vi "generic_test_noTEC.vi"() -> ()   [LabVIEW 2011]
uses:
  C:/OmniDriverSPAM/OOI_HOME/NETOmniDriver-NET20.dll
  OmniDriverSPAM/OOI_HOME/NETOmniDriver-NET20.dll
panel:
  out "getSpectrum Times Array":u32[](array[numeric])
  in  "ExtraDelay\nAfter Loop":bool
  in  "LoopExit":bool
  out "getSpectrumTime [ms]":u32
  in  "Trigger Mode":i32
  out "Spectrometer Type":string
  out "XY Graph":cluster{"Y":dbl[], "Y":dbl[]}[](graph) caption="XY-Graph"
  out "Spectrum":dbl[](array[numeric])
  out "Wavelengths [nm]":dbl[](array[numeric])
  in  "Scans to Average":i32=1
  in  "Int. Time [ms]":i32=1000
  out "MinIntTime [ms]":i32
  out "NETWrapper\nStatus":errorcluster caption="NETWrapper Status"
  out "MaxIntTime [ms]":i32
  in  "spectrometerIndex":i32
  out "Serial\nNumber":string
  out "Number attached\nSpectrometers":i32
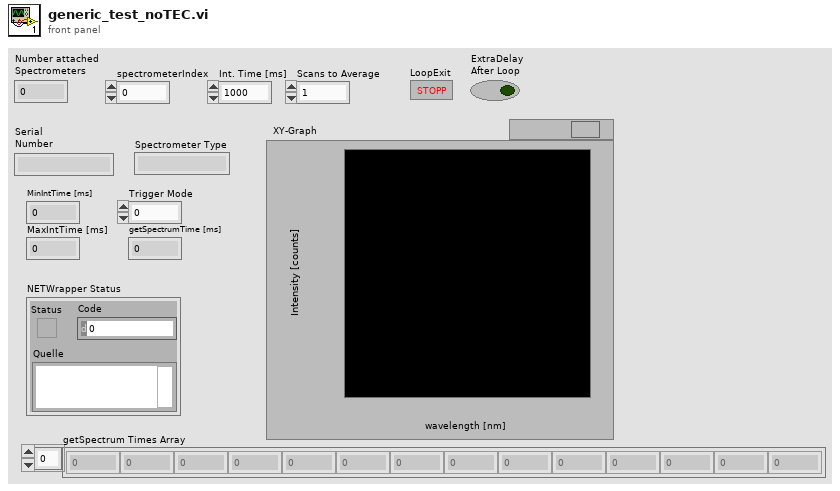
[diagram p1: front panel]
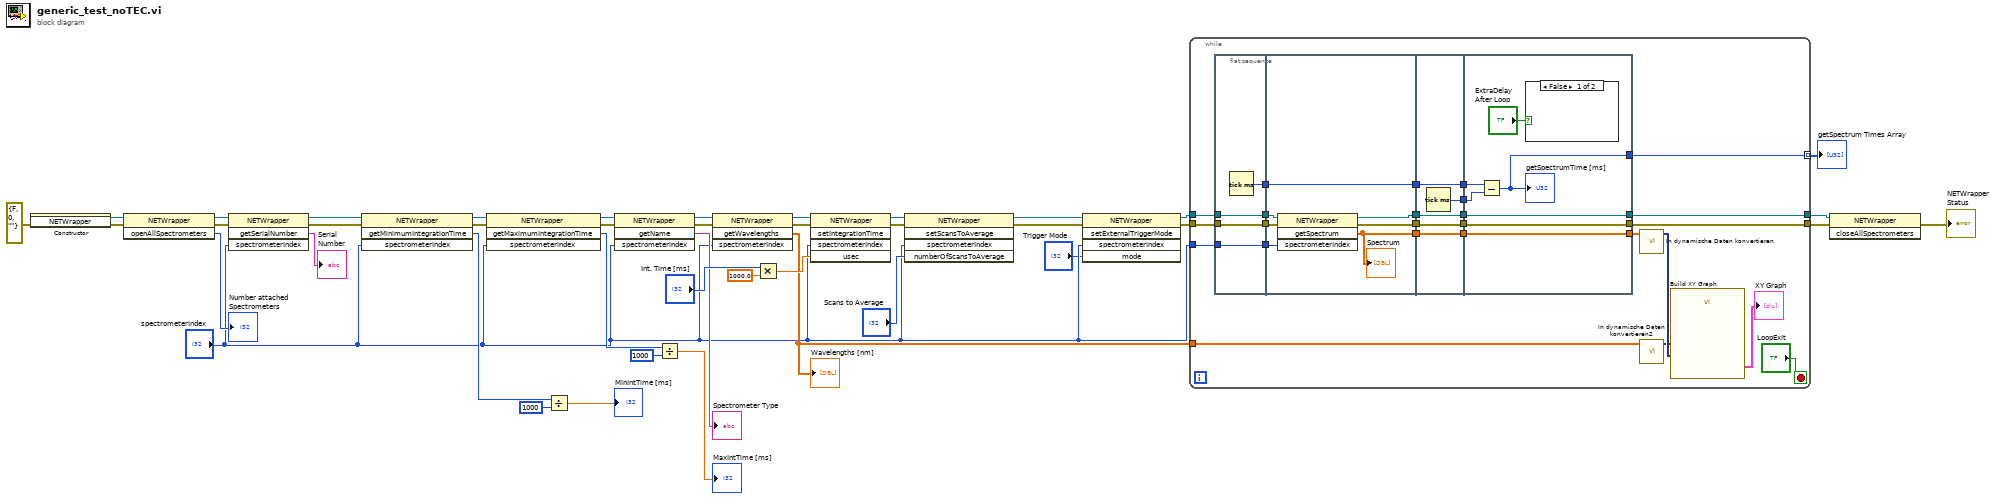
[diagram p0: block diagram]
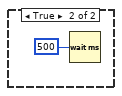
[diagram p2: hidden frame]
diagram:
  n1 = constructor class="NETWrapper"(error in=errorcluster {"status"=FALSE, "code"=0, "source"=""} ("Fehler (Eingang, kein Fehler)")) -> (reference out=w3:refnum<k24>, error out=w2:errorcluster)  [unwired: 2 in, 1 out]
  n2 = invoke class="NETWrapper" method="openAllSpectrometers"(reference=w3, error in=w2) -> (reference out=w40:refnum<k24>, error out=w39:errorcluster, "openAllSpectrometers"=→"Number attached\nSpectrometers":i32)  [unwired: 1 in]
  n3 = invoke class="NETWrapper" method="getSerialNumber"(reference=w40, error in=w39, "spectrometerIndex"="spectrometerIndex") -> (reference out=w37:refnum<k24>, error out=w36:errorcluster, "getSerialNumber"=→"Serial\nNumber":string)  [unwired: 1 in, 1 out]
  n4 = invoke class="NETWrapper" method="getMinimumIntegrationTime"(reference=w37, error in=w36, "spectrometerIndex"="spectrometerIndex") -> (reference out=w35:refnum<k24>, error out=w34:errorcluster, "getMinimumIntegrationTime"=w30:i32)  [unwired: 1 in, 1 out]
  n5 = invoke class="NETWrapper" method="getMaximumIntegrationTime"(reference=w35, error in=w34, "spectrometerIndex"="spectrometerIndex") -> (reference out=w14:refnum<k24>, error out=w16:errorcluster, "getMaximumIntegrationTime"=w15:i32)  [unwired: 1 in, 1 out]
  n6 = Divide(x=w30, y=1000) -> (x/y=→"MinIntTime [ms]":dbl)
  n7 = invoke class="NETWrapper" method="getName"(reference=w14, error in=w16, "spectrometerIndex"="spectrometerIndex") -> (reference out=w12:refnum<k24>, error out=w11:errorcluster, "getName"=→"Spectrometer Type":string)  [unwired: 1 in, 1 out]
  n8 = Divide(x=w15, y=1000) -> (x/y=→"MaxIntTime [ms]":dbl)
  n9 = invoke class="NETWrapper" method="getWavelengths"(reference=w12, error in=w11, "spectrometerIndex"="spectrometerIndex") -> (reference out=w21:refnum<k24>, error out=w20:errorcluster, "getWavelengths"=w17:dbl[])  [unwired: 1 in, 1 out]
  "Wavelengths [nm]" <- w17
  n10 = Multiply(x="Int. Time [ms]", y=1000.0) -> (x*y=w27:dbl)
  n11 = invoke class="NETWrapper" method="setIntegrationTime"(reference=w21, error in=w20, "spectrometerIndex"="spectrometerIndex", "usec"=w27) -> (reference out=w23:refnum<k24>, error out=w24:errorcluster)  [unwired: 1 in, 3 out]
  n12 = invoke class="NETWrapper" method="setScansToAverage"(reference=w23, error in=w24, "spectrometerIndex"="spectrometerIndex", "numberOfScansToAverage"="Scans to Average") -> (reference out=w9:refnum<k24>, error out=w8:errorcluster)  [unwired: 1 in, 3 out]
  n13 = invoke class="NETWrapper" method="setExternalTriggerMode"(reference=w9, error in=w8, "spectrometerIndex"="spectrometerIndex", "mode"="Trigger Mode") -> (reference out=w10:refnum<k24>, error out=w7:errorcluster)  [unwired: 1 in, 3 out]
  n14 = while {
    tunnel: w10 -> [w66]
    tunnel: [w65] -> w19
    tunnel: [w64] -> w18
    tunnel: w17 -> [w60]
    tunnel: "spectrometerIndex" -> [w58]
    tunnel: w7 -> [w57]
    tunnel: [w42] -> w4 mode=indexing
    stop <- "LoopExit" stop-if-true
    n15 = flat-sequence {
      tunnel: w57 -> [w68]
      tunnel: w58 -> [w69]
      tunnel: w66 -> [w70]
      tunnel: [w70] -> w56
      tunnel: [w69] -> w55
      tunnel: [w68] -> w54
      tunnel: [w67] -> w46
      tunnel: w56 -> [w77]
      tunnel: w55 -> [w74]
      tunnel: w54 -> [w73]
      tunnel: [w76] -> w53
      tunnel: [w75] -> w52
      tunnel: [w72] -> w51
      tunnel: w46 -> [w71]
      tunnel: [w71] -> w45
      tunnel: w53 -> [w82]
      tunnel: w52 -> [w81]
      tunnel: w51 -> [w80]
      tunnel: [w82] -> w50
      tunnel: [w81] -> w49
      tunnel: [w80] -> w48
      tunnel: [w79] -> w47
      tunnel: w45 -> [w78]
      tunnel: [w78] -> w44
      tunnel: [w87] -> w62
      tunnel: [w88] -> w64
      tunnel: [w89] -> w65
      tunnel: w50 -> [w89]
      tunnel: w49 -> [w88]
      tunnel: w48 -> [w87]
      tunnel: w47 -> [w86]
      tunnel: w44 -> [w85]
      tunnel: [w83] -> w42
      frame #0 {
        n16 = Tick Count (ms)() -> (millisecond timer value=w67:u32)
      }
      frame #1 {
        n17 = invoke class="NETWrapper" method="getSpectrum"(reference=w77, error in=w73, "spectrometerIndex"=w74) -> (reference out=w76:refnum<k24>, error out=w75:errorcluster, "getSpectrum"=w72:dbl[])  [unwired: 1 in, 1 out]
        "Spectrum" <- w72
      }
      frame #2 {
        n18 = Tick Count (ms)() -> (millisecond timer value=w79:u32)
      }
      frame #3 {
        n19 = Subtract(x=w85, y=w86) -> (x-y=w83:u32)
        "getSpectrumTime [ms]" <- w83
        n20 = case shown="False" "ExtraDelay\nAfter Loop" {
          frame False {
          }
          frame True {
            n21 = Wait (ms)(milliseconds to wait=u32 500 ("Zu wartende ms")) -> ()  [unwired: 1 out]
          }
        }
      }
    }
    n22 = call "In dynamische Daten konvertieren"("Array"=w62) -> ("Dynamic Data Type"=w61:dynamicdata)  [unwired: 3 in]
    n23 = call "In dynamische Daten konvertieren2"("Array"=w60) -> ("Dynamic Data Type"=w59:dynamicdata)  [unwired: 3 in]
    n24 = call "Build XY Graph"("Y Input"=w61, "X Input"=w59) -> ("XY Graph"=→"XY Graph":cluster{"Y":dbl[], "Y":dbl[]}[])  [unwired: 3 in, 6 out]
  }
  "getSpectrum Times Array" <- w4
  n25 = invoke class="NETWrapper" method="closeAllSpectrometers"(reference=w19, error in=w18) -> (error out=→"NETWrapper\nStatus":errorcluster)  [unwired: 1 in, 2 out]
